vi "Pointer.Read (U8).vi"(8 "error in (no error)":errorcluster, 11 "pointer in":u64) -> (0 "error out":errorcluster, 2 "value":u8, 3 "pointer out":u64)   [LabVIEW 2016, in "VeriStand Data.lvlib"]
doc: "Read a value from the provided <B>pointer</B>."
uses:
  VeriStand Data.lvlib
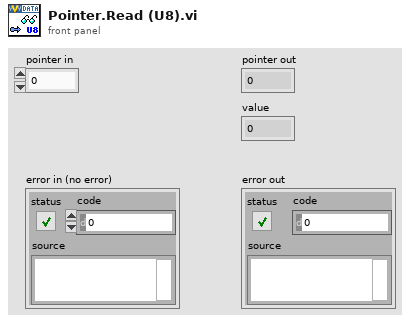
[diagram p1: front panel]
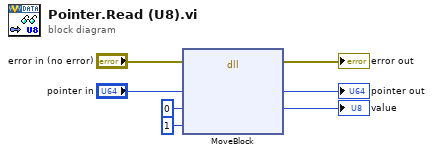
[diagram p0: block diagram]
diagram:
  n1 = dll-call lib="LabVIEW" fn="MoveBlock"(error in="error in (no error)", "ps"="pointer in", "pd"=u8 0, "size"=u64 1) -> (error out=→"error out":errorcluster, "ps"=→"pointer out":u64, "pd"=→"value":u8)  [unwired: 4 in, 1 out]
